vi "Initialize.vi"(8 "error in":errorcluster, 10 "parameters":variant, 11 "node in":refnum<class "NISE_CEF_serializable node.lvclass">) -> (0 "error out":errorcluster, 2 "summary":T2[](array[typedef]), 3 "data value reference":T1)   [LabVIEW 2013, in "NISE_CEF_serializable node.lvclass"]
doc: "Initializes the data of a node to its default state.\nThe object is not created inside of this VI, because it is created from a File depending on user selection."
uses:
  NISE_CEF_serializable node.lvclass
  Node/NISE_CEF_Node.lvclass
  serializable configuration/NISE_CEF_serializable configuration.lvclass
  Node/Summary.ctl
  Node/NodeRef.ctl
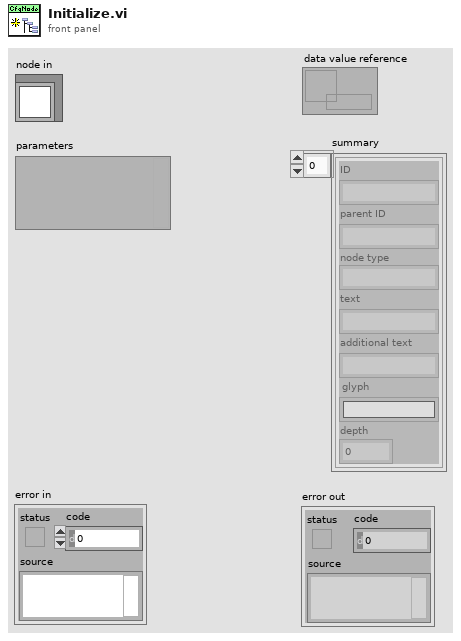
[diagram p1: front panel]
types:
  T1 = typedef "NISE_CEF_Node.lvclass/NodeRef.ctl" = refnum<data-value>
  T2 = typedef "NISE_CEF_Node.lvclass/Summary.ctl" = cluster{"ID":string, "parent ID":string, "node type":string, "text":string, "additional text":string, "glyph":string, "depth":i32}
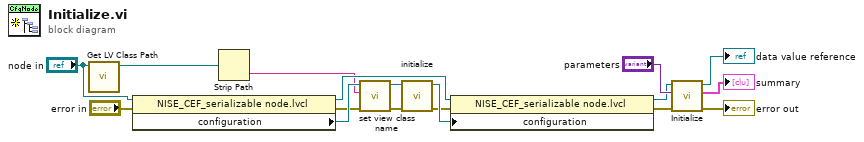
[diagram p0: block diagram]
diagram:
  n1 = call <vilib>:"Get LV Class Path.vi"("object"="node in") -> ("class path"=w2:path)  [unwired: 9 in, 1 out]
  n2 = property class="NISE_CEF_serializable node.lvcl"(reference="node in", error in="error in") -> (reference out=w10:refnum<class "NISE_CEF_serializable node.lvclass">, error out=w4:errorcluster, "configuration"=w7:refnum<class "NISE_CEF_serializable configuration.lvclass">)
  n3 = Strip Path(path=w2) -> (name=w1:string)  [unwired: 1 out]
  n4 = call "set view class name.vi"("error in"=w4, "view class"=w1, "configuration in"=w7) -> ("error out"=w5:errorcluster, "configuration out"=w6:refnum<class "NISE_CEF_serializable configuration.lvclass">)  [unwired: 7 in]
  n5 = call-dynamic "initialize.vi"("error in"=w5, "configuration in"=w6) -> ("error out"=w8:errorcluster, "configuration out"=w9:refnum<class "NISE_CEF_serializable configuration.lvclass">)  [unwired: 7 in, 1 out]
  n6 = property class="NISE_CEF_serializable node.lvcl"(reference=w10, error in=w8, "configuration"=w9) -> (reference out=w11:refnum<class "NISE_CEF_serializable node.lvclass">, error out=w12:errorcluster)
  n7 = call-parent "Initialize.vi"("error in"=w12, "parameters"="parameters", "node in"=w11) -> ("error out"=→"error out":errorcluster, "summary"=→"summary":T2[], "data value reference"=→"data value reference":T1)  [unwired: 6 in]
